vi "Do.vi"(8 "error in (no error)":errorcluster, 10 "Actor in":refnum<class "Actor.lvclass">, 11 "Update Array Msg":refnum<class "Update Boolean Event Msg.lvclass">) -> (0 "error out":errorcluster, 2 "Actor out":refnum<class "Actor.lvclass">)   [LabVIEW 2023, in "Example MVC Actors.lvlib" / "Example View.lvlib" / "Update Boolean Event Msg.lvclass"]
doc: "This VI delivers the message to the actor by calling the appropriate method(s) on the actor."
uses:
  Update Boolean Event Msg.lvclass
  C:/Projects/Shared Libraries/Event Actors/Event Handlers/Abstract Event Message for View/Abstract Event Message for View.lvclass
  <vilib>/ActorFramework/Actor/Actor.lvclass
  Example View/Example View.lvclass
  C:/Program Files/National Instruments/LabVIEW 2023/vi.lib/ActorFramework/Actor/Actor.lvclass
  Example Events/Boolean Event.lvclass
  C:/Projects/Shared Libraries/Event Actors/Event Data Types/Event Boolean/Event Boolean.lvclass
  Event Handlers/Abstract Event Message for View/Abstract Event Message for View.lvclass/Abstract Event Message for View.ctl
  Event Handlers/Abstract Event Message for View/Abstract Event Message for View.lvclass
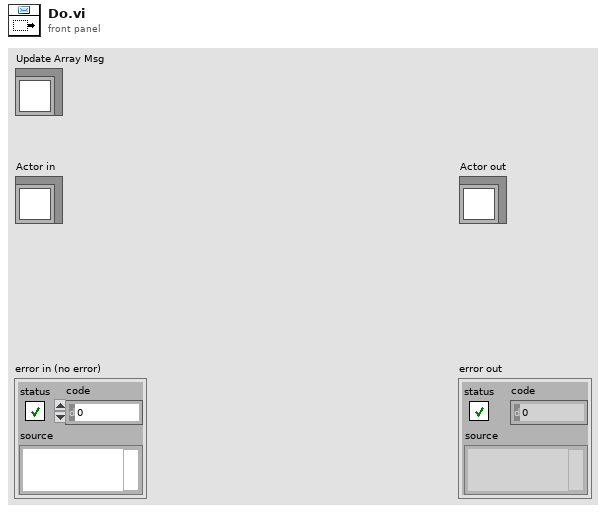
[diagram p1: front panel]
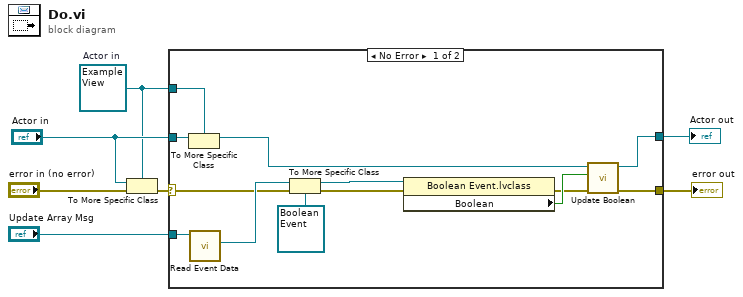
[diagram p0: block diagram]
diagram:
  w2 = refnum<class "Example View.lvclass"> refnum  # Actor in
  n1 = To More Specific Class(target class=w2, reference="Actor in", error in="error in (no error)") -> (error out=w1:errorcluster)  [unwired: 1 out]
  n2 = case shown="No Error" w1 {
    selector: w1 -> [w10 w22]
    tunnel: [w20 w22] -> w7
    tunnel: [w19 w21] -> w6
    tunnel: "Actor in" -> [w18 w21]
    tunnel: w2 -> [w17 _]
    tunnel: "Update Array Msg" -> [w14 _]
    frame No Error {
      n3 = To More Specific Class(target class=w17, reference=w18) -> (specific class reference=w16:refnum<class "Example View.lvclass">)  [unwired: 1 in, 1 out]
      n4 = call "Read Event Data.vi"("Event Generated Msg"=w14) -> ("Event Data"=w13:refnum<class "Event.lvclass">)  [unwired: 10 in]
      n5 = To More Specific Class(target class=refnum<class "Boolean Event.lvclass"> refnum ("Example Source.lvlib:Boolean Event.lvclass"), reference=w13, error in=w10) -> (specific class reference=w12:refnum<class "Boolean Event.lvclass">, error out=w9:errorcluster)
      n6 = property class="Boolean Event.lvclass"(reference=w12, error in=w9) -> (error out=w8:errorcluster, "Boolean"=w11:bool)  [unwired: 1 out]
      n7 = call "Update Boolean.vi"("error in (no error)"=w8, "Boolean"=w11, "Example View in"=w16) -> ("error out"=w20:errorcluster, "Example View out"=w19:refnum<class "Example View.lvclass">)  [unwired: 7 in]
    }
    frame Error {
      # "If type check fails, pass the original object out again."
    }
  }
  "error out" <- w7
  "Actor out" <- w6
